vi "test read reg.vi"() -> ()   [LabVIEW 2019]
uses:
  <vilib>/registry/registry.llb/Registry SAM.ctl
  <vilib>/registry/registry.llb/Read Registry Value Simple STR.vi
  <vilib>/regexp/Match Regular Expression.xnode
panel:
  in  "error in (no error)":errorcluster
  out "error out":errorcluster
  out "ComPort":string[](array[string])
  out "Serial Number":string[](array[string])
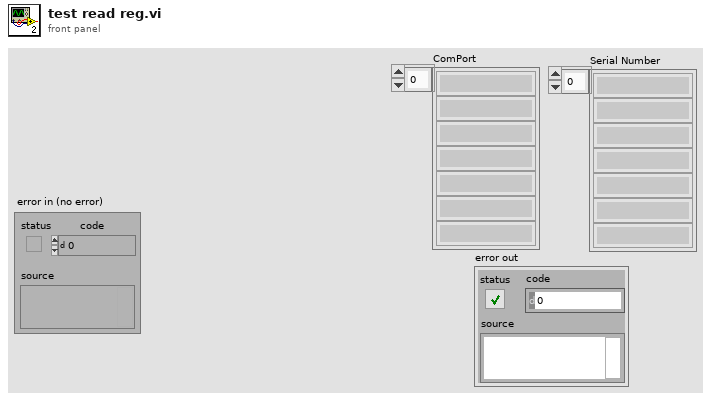
[diagram p1: front panel]
types:
  T1 = typedef "Registry SAM.ctl" = enum32{"KEY_QUERY_VALUE", "KEY_SET_VALUE", "KEY_CREATE_SUB_KEY", "KEY_ENUMERATE_SUB_KEYS", "KEY_NOTIFY", "KEY_CREATE_LINK", "KEY_READ", "KEY_WRITE", "KEY_ALL_ACCESS", "KEY_READ | KEY_WRITE"}
  T2 = typedef "Registry refnum.ctl" = refnum<k1>
  T3 = cluster{"numSubKeys":i32, "maxSubKeyLen":i32, "maxSubKeyClassLen":i32}
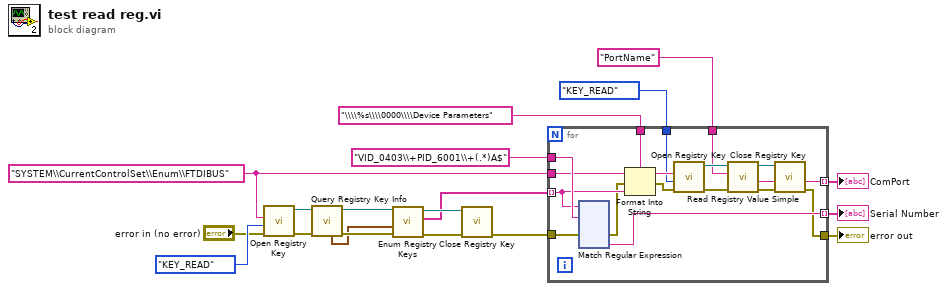
[diagram p0: block diagram]
diagram:
  w9 = "SYSTEM\\CurrentControlSet\\Enum\\FTDIBUS" ("subkey")
  n1 = call <vilib>:"Open Registry Key.vi"("error in (no error)"="error in (no error)", "security access mask (KEY_READ | KEY_WRITE)"=Registry_SAM."KEY_READ", "subkey"=w9) -> ("error out"=w17:errorcluster, "refnum out"=w19:T2)  [unwired: 7 in]
  n2 = call <vilib>:"Query Registry Key Info.vi"("error in (no error)"=w17, "refnum"=w19) -> ("error out"=w16:errorcluster, "refnum out"=w18:T2, "subkey info"=w14:T3)  [unwired: 5 in, 2 out]
  n3 = call <vilib>:"Enum Registry Keys.vi"("error in (no error)"=w16, "subkey info"=w14, "refnum"=w18) -> ("error out"=w4:errorcluster, "subkeys"=w12:string[], "refnum out"=w13:T2)  [unwired: 6 in]
  n4 = call <vilib>:"Close Registry Key.vi"("error in (no error)"=w4, "refnum"=w13) -> ("error out"=w2:errorcluster)  [unwired: 5 in]
  n5 = for {
    tunnel: w12 -> [w33] mode=indexing
    tunnel: "VID_0403\\+PID_6001\\+(.*)A$" ("regular expression") -> [w36]
    tunnel: [w35] -> w10 mode=indexing
    tunnel: w9 -> [w34]
    tunnel: Registry_SAM."KEY_READ" ("security access mask (KEY_READ | KEY_WRITE)") -> [w30]
    tunnel: "\\\\%s\\\\0000\\\\Device Parameters" ("regular expression") -> [w29]
    tunnel: "PortName" ("value") -> [w27]
    tunnel: [w26] -> w5 mode=indexing
    tunnel: w2 -> [w23]
    tunnel: [w20] -> w1
    n6 = xnode "Match Regular Expression"("input string"=w33, "regular expression"=w36, "error in"=w23) -> ("error out"=w22:errorcluster, "submatch 1"=w35:string)  [unwired: 3 in, 4 out]
    n7 = Format Into String(format string=w29, initial string=w34, error in=w22, w33) -> (resulting string=w32:string, error out=w21:errorcluster)
    n8 = call <vilib>:"Open Registry Key.vi"("error in (no error)"=w21, "security access mask (KEY_READ | KEY_WRITE)"=w30, "subkey"=w32) -> ("error out"=w28:errorcluster, "refnum out"=w31:T2)  [unwired: 7 in]
    n9 = call-poly <vilib>:"Read Registry Value Simple.vi"("error in (no error)"=w28, "value"=w27, "refnum"=w31) -> ("error out"=w25:errorcluster, "String/Binary data"=w26:string, "refnum out"=w24:T2)  [unwired: 3 in, 1 out]
    n10 = call <vilib>:"Close Registry Key.vi"("error in (no error)"=w25, "refnum"=w24) -> ("error out"=w20:errorcluster)  [unwired: 5 in]
  }
  "Serial Number" <- w10
  "ComPort" <- w5
  "error out" <- w1
